vi "汇总单个量测项目数据.vi"(10 "精度(6)":i16=3, 11 "测量数值":dbl[](array[numeric])) -> (3 "单个量测项目结果":string)   [LabVIEW 2014]
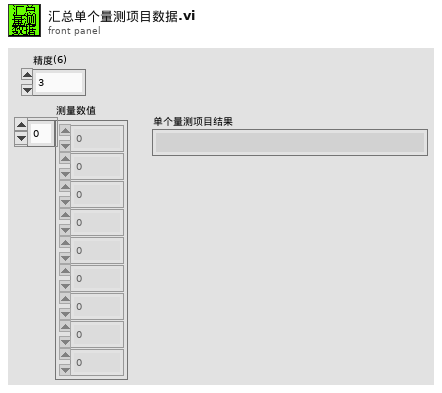
[diagram p1: front panel]
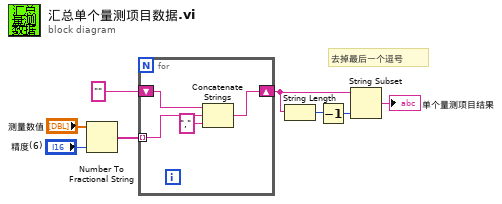
[diagram p0: block diagram]
diagram:
  # "去掉最后一个逗号"
  n1 = Number To Fractional String(number="测量数值", precision (6)="精度(6)") -> (F-format string=w7:string[])  [unwired: 2 in]
  n2 = for {
    tunnel: w7 -> [w11] mode=indexing
    shift-right: [w9] -> w4
    shift-left: "" -> [w12]
    n3 = Concatenate Strings(w12, w11, "," ("字符串")) -> (w9:string)
  }
  n4 = String Length(string=w4) -> (length=w3:i32)
  n5 = Decrement(x=w3) -> (x-1=w2:i32)
  n6 = String Subset(string=w4, length (rest)=w2) -> (substring=→"单个量测项目结果":string)  [unwired: 1 in]
